vi "SW_Load_parameter_group.vi"(7 "Settings file refnum in":T1, 8 "error in":errorcluster, 9 "Default value (JSON)":string, 10 "Group":string, 11 "Researcher name":string) -> (0 "error out":errorcluster, 2 "Read value (JSON)":string, 3 "Settings file refnum out":T1)   [LabVIEW 2018]
uses:
  <vilib>/Utility/config.llb/Config Data RefNum.ctl
  <vilib>/Utility/config.llb/Read Key (String).vi
  <vilib>/Utility/config.llb/Write Key (String).vi
  <vilib>/Utility/config.llb/NI_LVConfig.lvlib
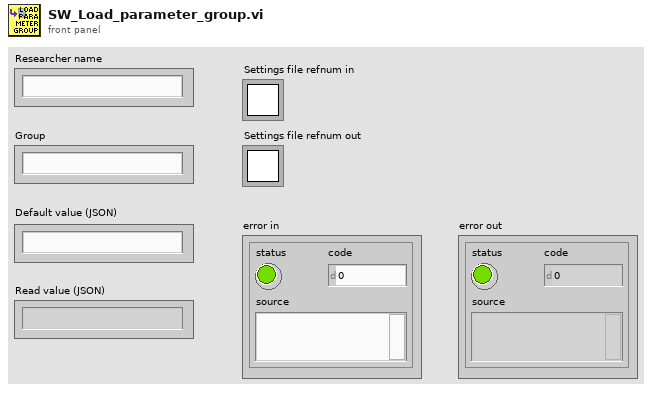
[diagram p1: front panel]
types:
  T1 = typedef "NI_LVConfig.lvlib/Config Data RefNum.ctl" = refnum<k1>
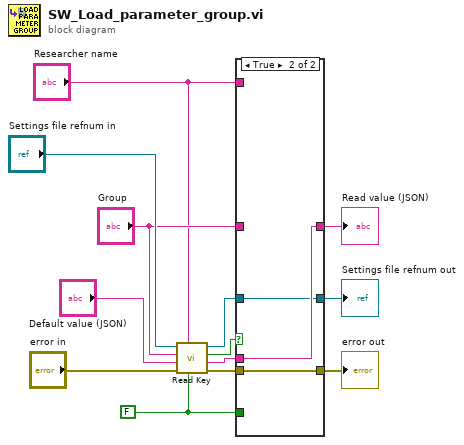
[diagram p0: block diagram]
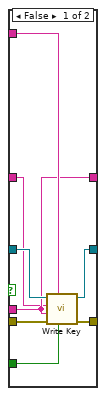
[diagram p2: hidden frame]
diagram:
  w5 = FALSE ("read raw string? (F)")
  n1 = call-poly <vilib>:"Read Key.vi"("read raw string? (F)"=w5, "section"="Researcher name", "error in (no error)"="error in", "default value"="Default value (JSON)", "key"="Group", "refnum"="Settings file refnum in") -> ("error out"=w9:errorcluster, "value"=w8:string, "found?"=w11:bool, "refnum out"=w10:T1)  [unwired: 2 in]
  n2 = case shown="True" w11 {
    tunnel: w10 -> [w21 w22]
    tunnel: w9 -> [w20 w23]
    tunnel: w8 -> [w15 w24]
    tunnel: "Researcher name" -> [w19 _]
    tunnel: w5 -> [w18 _]
    tunnel: [w17 w23] -> w7
    tunnel: [w16 w22] -> w2
    tunnel: [w15 w24] -> w6
    tunnel: "Group" -> [w14 _]
    frame False {
      n3 = call-poly <vilib>:"Write Key.vi"("write raw string? (F)"=w18, "section"=w19, "error in (no error)"=w20, "value"=w15, "key"=w14, "refnum"=w21) -> ("error out"=w17:errorcluster, "refnum out"=w16:T1)  [unwired: 3 in, 1 out]
    }
    frame True {
    }
  }
  "error out" <- w7
  "Read value (JSON)" <- w6
  "Settings file refnum out" <- w2
